vi "test_OneSessTwoPinOneSystemPinOneInstrOneSiteReservation_CallGetConnectionsFromPinsForTwoDcPowerPinsAllSites_ReturnsTwoConnections.vi"(8 "error in":errorcluster) -> (0 "error out":errorcluster, 2 "result":string, 3 "pass":bool)   [LabVIEW 2020, in "MeasurementServerTests.lvlib"]
uses:
  MeasurementServerTests.lvlib
  Runtime/MeasurementLink Session Management V1/Session Reservation/Connection.ctl
  Runtime/MeasurementLink Session Management V1/Session Reservation/Session Reservation.lvclass
  Runtime/MeasurementLink Session Management V1/Session Reservation/Connection with Session.ctl
  b3e5c3be-b7a7-4b6e-86ee-709eea9cb752.vi
  c3cb69a0-23cd-49fc-99d1-8c54773f0200.vi
  777eb16d-c0be-4c50-a7a6-d4611c66469e.vi
  Runtime/MeasurementLink niDCPower/Session Factory/Session Factory.lvclass
  54d890a8-4121-421c-bfc5-08266fe71a04.vi
  Runtime/MeasurementLink Session Management V1/Session Reservation/Pin Type.ctl
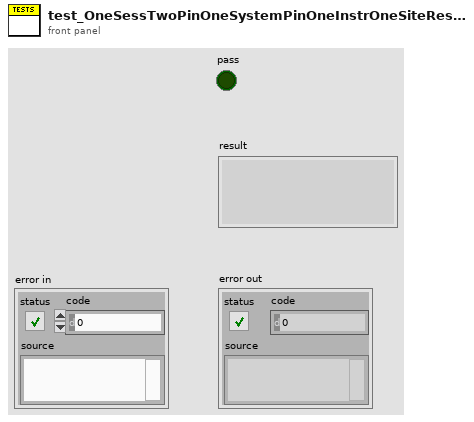
[diagram p1: front panel]
types:
  T1 = typedef "MeasurementLink Session Management V1.lvlib/Session Reservation.lvclass/Pin Type.ctl" = enum16{"DUT and System Pins", "System Pins"}
  T2 = typedef "MeasurementLink Session Management V1.lvlib/Session Reservation.lvclass/Connection.ctl" = cluster{"pin or relay name":string, "site":i32, "instrument type id":string, "channel":string}
  T3 = typedef "MeasurementLink Session Management V1.lvlib/Session Reservation.lvclass/Connection with Session.ctl" = cluster{"connection":T2, "session":variant}
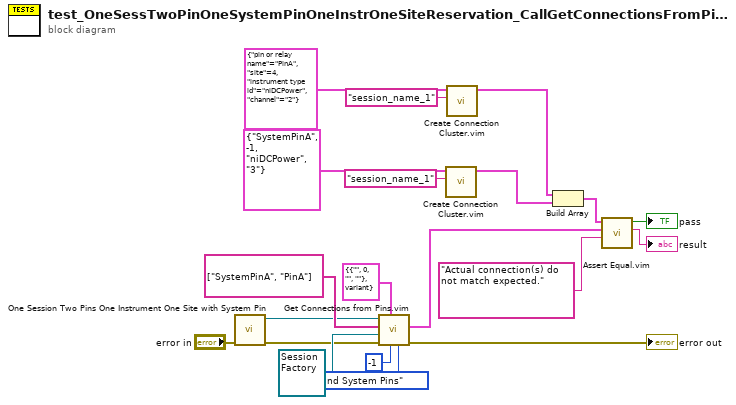
[diagram p0: block diagram]
diagram:
  n1 = call "One Session Two Pins One Instrument One Site with System Pin.vi"("error in"="error in") -> ("error out"=w1:errorcluster, "session reservation out"=w2:refnum<class "Session Reservation.lvclass">)  [unwired: 9 in]
  n2 = call "Get Connections from Pins.vim"("pin type"=Pin_Type."DUT and System Pins", "site"=-1, "connection type"=T3 {"connection"={"pin or relay name"="", "site"=0, "instrument type id"="", "channel"=""}, "session"=variant} ("connection"), "error in"=w1, "session factory"=refnum<class "Session Factory.lvclass"> refnum ("MeasurementLink niDCPower.lvlib:Instrument.lvclass"), "pin or relay names"=string[] ["SystemPinA", "PinA"], "session reservation in"=w2) -> ("error out"=→"error out":errorcluster, "connections"=w17:T3[])  [unwired: 2 in, 1 out]
  n3 = call "Create Connection Cluster.vim"("session in"="session_name_1", "hardware independent connection in"=T2 {"pin or relay name"="SystemPinA", "site"=-1, "instrument type id"="niDCPower", "channel"="3"} ("connection")) -> ("connection out"=w12:T3)  [unwired: 9 in]
  n4 = call "Create Connection Cluster.vim"("session in"="session_name_1", "hardware independent connection in"=T2 {"pin or relay name"="PinA", "site"=4, "instrument type id"="niDCPower", "channel"="2"} ("connection")) -> ("connection out"=w4:T3)  [unwired: 9 in]
  n5 = Build Array(w4, w12) -> (w11:T3[])
  n6 = call "Assert Equal.vim"("failure message"="Actual connection(s) do not match expected.", "actual value"=w17, "expected value"=w11) -> ("message"=→"result":string, "equal?"=→"pass":bool)  [unwired: 7 in]
